vi "ReadIni.vi"(1 "configuration file path":path) -> ()   [LabVIEW 2018]
uses:
  <vilib>/Utility/config.llb/Read Key (String).vi
  <vilib>/Utility/config.llb/NI_LVConfig.lvlib
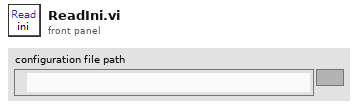
[diagram p1: front panel]
types:
  T1 = typedef "NI_LVConfig.lvlib/Config Data RefNum.ctl" = refnum<k1>
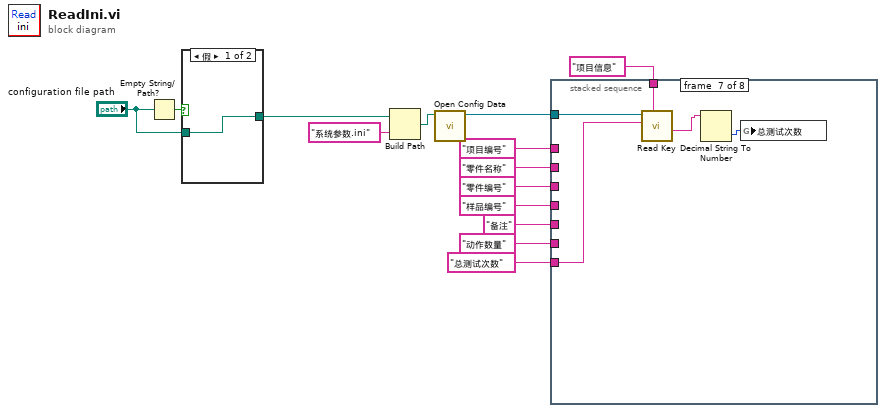
[diagram p0: block diagram]
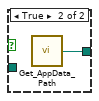
[diagram p2: hidden frame]
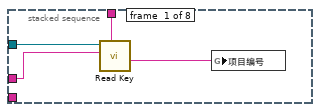
[diagram p3: hidden frame]
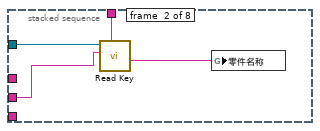
[diagram p4: hidden frame]
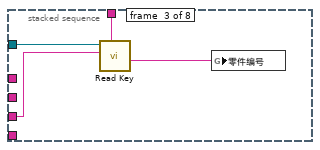
[diagram p5: hidden frame]
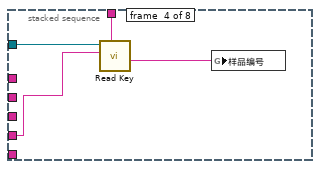
[diagram p6: hidden frame]
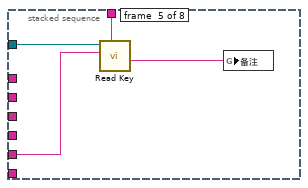
[diagram p7: hidden frame]
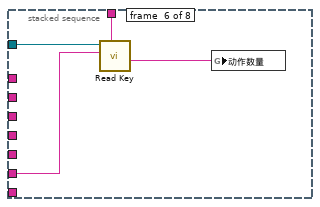
[diagram p8: hidden frame]
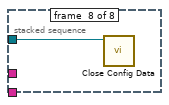
[diagram p9: hidden frame]
diagram:
  n1 = Empty String/Path?(string/path="configuration file path") -> (empty?=w4:bool)
  n2 = case shown="假" w4 {
    tunnel: [w15 w16] -> w3
    tunnel: "configuration file path" -> [w15 _]
    frame False {
    }
    frame True {
      n3 = call "Get_AppData_Path.vi"() -> ("path"=w16:path)  [unwired: 1 in]
    }
  }
  n4 = Build Path(base path=w3, name or relative path="系统参数.ini" ("名称或相对路径")) -> (appended path=w14:path)
  n5 = call <vilib>:"Open Config Data.vi"("configuration file path"=w14) -> ("refnum"=w12:T1)  [unwired: 8 in, 2 out]
  n6 = stacked-sequence {
    tunnel: w12 -> [w19 w23 w27 w31 w35 w39 w45 w46]
    tunnel: "项目信息" -> [w18 w22 w26 w30 w34 w38 w41 _]
    tunnel: "零件名称" -> [_ w21 _ _ _ _ _ _]
    tunnel: "项目编号" -> [w17 _ _ _ _ _ _ _]
    tunnel: "零件编号" -> [_ _ w25 _ _ _ _ _]
    tunnel: "样品编号" -> [_ _ _ w29 _ _ _ _]
    tunnel: "备注" -> [_ _ _ _ w33 _ _ _]
    tunnel: "动作数量" -> [_ _ _ _ _ w37 _ _]
    tunnel: "总测试次数" -> [_ _ _ _ _ _ w44 _]
    frame #0 {
      n7 = call-poly <vilib>:"Read Key.vi"("section"=w18, "key"=w17, "refnum"=w19) -> ("value"=w20:string)  [unwired: 5 in, 3 out]
      n8 = global write "全局 1.vi" "项目编号"(w20) -> ()
    }
    frame #1 {
      n9 = call-poly <vilib>:"Read Key.vi"("section"=w22, "key"=w21, "refnum"=w23) -> ("value"=w24:string)  [unwired: 5 in, 3 out]
      n10 = global write "全局 1.vi" "零件名称"(w24) -> ()
    }
    frame #2 {
      n11 = call-poly <vilib>:"Read Key.vi"("section"=w26, "key"=w25, "refnum"=w27) -> ("value"=w28:string)  [unwired: 5 in, 3 out]
      n12 = global write "全局 1.vi" "零件编号"(w28) -> ()
    }
    frame #3 {
      n13 = call-poly <vilib>:"Read Key.vi"("section"=w30, "key"=w29, "refnum"=w31) -> ("value"=w32:string)  [unwired: 5 in, 3 out]
      n14 = global write "全局 1.vi" "样品编号"(w32) -> ()
    }
    frame #4 {
      n15 = call-poly <vilib>:"Read Key.vi"("section"=w34, "key"=w33, "refnum"=w35) -> ("value"=w36:string)  [unwired: 5 in, 3 out]
      n16 = global write "全局 1.vi" "备注"(w36) -> ()
    }
    frame #5 {
      n17 = call-poly <vilib>:"Read Key.vi"("section"=w38, "key"=w37, "refnum"=w39) -> ("value"=w40:string)  [unwired: 5 in, 3 out]
      n18 = global write "全局 1.vi" "动作数量"(w40) -> ()
    }
    frame #6 {
      n19 = call-poly <vilib>:"Read Key.vi"("section"=w41, "key"=w44, "refnum"=w45) -> ("value"=w42:string)  [unwired: 5 in, 3 out]
      n20 = Decimal String To Number(string=w42) -> (number=w43:i32)  [unwired: 2 in, 1 out]
      n21 = global write "全局 1.vi" "总测试次数"(w43) -> ()
    }
    frame #7 {
      n22 = call <vilib>:"Close Config Data.vi"("refnum"=w46) -> ()  [unwired: 9 in, 2 out]
    }
  }
